vi "Update Logic Outputs.vi"(8 "error in (no error)":errorcluster, 10 "Array of LogicIO POWER OFF":bool[](array[boolean]), 11 "VacuumLine in":refnum<class "VacuumLine.lvclass">) -> (0 "error out":errorcluster, 3 "VacuumLine out":refnum<class "VacuumLine.lvclass">)   [LabVIEW 2016, in "Hardware.lvlib" / "VacuumLine.lvlib" / "VacuumLine.lvclass"]
uses:
  <userlib>/Common Components/Hardware/Abstract System/VacuumLine/VacuumLine/VacuumLine.lvclass
  <userlib>/Common Components/Hardware/Abstract System/VacuumLine/VacuumLine/VacuumLine.lvclass/VacuumLine.ctl
  <userlib>/Common Components/Hardware/LogicIO/LogicIO/LogicIO.lvclass
  C:/Program Files (x86)/National Instruments/LabVIEW 2016/user.lib/Common Components/Hardware/Abstract Hardware/Hardware.lvclass
  <vilib>/Utility/error.llb/Error Cluster From Error Code.vi
  <vilib>/ErrorRing/Error Ring.xnode
  <userlib>/Common Components/Hardware/Abstract Hardware/Hardware.lvclass
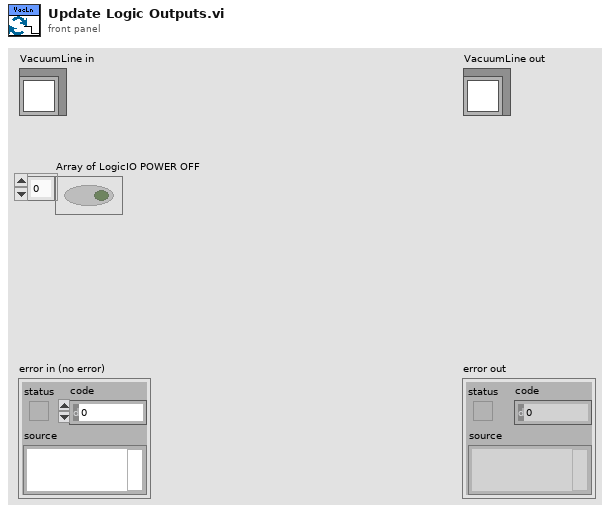
[diagram p1: front panel]
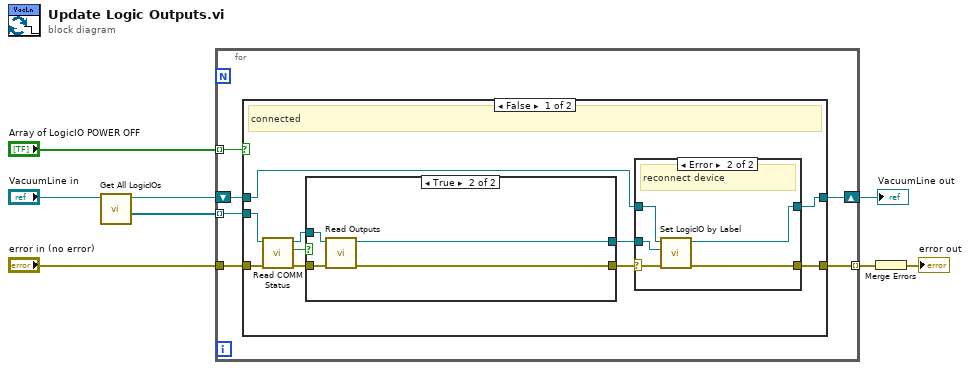
[diagram p0: block diagram]
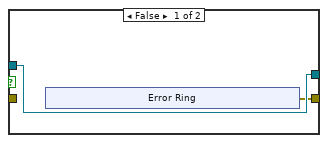
[diagram p2: hidden frame]
diagram:
  n1 = call <userlib>:"Get All LogicIOs.vi"("VacuumLine in"="VacuumLine in") -> ("LogicIOs"=w7:refnum<class "LogicIO.lvclass">[], "VacuumLine out"=w6:refnum<class "VacuumLine.lvclass">)  [unwired: 7 in, 2 out]
  n2 = for {
    tunnel: w7 -> [w14] mode=indexing
    shift-right: [w12] -> w5
    shift-left: w6 -> [w13]
    tunnel: [w10] -> w3 mode=indexing
    tunnel: "error in (no error)" -> [w11]
    tunnel: "Array of LogicIO POWER OFF" -> [w9] mode=indexing
    n3 = case shown="False" w9 {
      tunnel: w14 -> [w24 _]
      tunnel: w13 -> [w23 w43]
      tunnel: [w21 w43] -> w12
      tunnel: w11 -> [w17 w42]
      tunnel: [w19 w42] -> w10
      frame False {
        # "connected"
        n4 = call <userlib>:"Read COMM Status.vi"("error in (no error)"=w17, "Hardware in"=w24) -> ("error out"=w16:errorcluster, "COMM status"=w15:bool, "Hardware out"=w18:refnum<class "LogicIO.lvclass">)  [unwired: 7 in]
        n5 = case shown="True" w15 {
          tunnel: [w26 w34] -> w22
          tunnel: [w25 w33] -> w20
          tunnel: w18 -> [w26 w32]
          tunnel: w16 -> [_ w31]
          frame False {
            n6 = xnode "Error Ring"() -> ("error out"=w25:errorcluster)
          }
          frame True {
            n7 = call-dynamic "Read Outputs.vi"("error in (no error)"=w31, "LogicIO in"=w32) -> ("error out"=w33:errorcluster, "LogicIO out"=w34:refnum<class "LogicIO.lvclass">)  [unwired: 7 in, 1 out]
          }
        }
        n8 = case shown="Error" w20 {
          selector: w20 -> [w35 w38]
          tunnel: w23 -> [w36 w41]
          tunnel: w22 -> [_ w40]
          tunnel: [w36 w39] -> w21
          tunnel: [w35 w37] -> w19
          frame No Error {
          }
          frame Error {
            # "reconnect device"
            n9 = call <userlib>:"Set LogicIO by Label.vi"("error in (no error)"=w38, "LogicIO obj"=w40, "VacuumLine in"=w41) -> ("error out"=w37:errorcluster, "VacuumLine out"=w39:refnum<class "VacuumLine.lvclass">)  [unwired: 7 in]
          }
        }
      }
      frame True {
        # "powered off"
      }
    }
  }
  "VacuumLine out" <- w5
  n10 = Merge Errors(w3) -> (→"error out":errorcluster)
